vi "test cli options.vi"() -> ()   [LabVIEW 2024]
uses:
  <vilib>/Wiresmith Technology/G CLI/Argument Parser/Option Set Class/Option Set.lvclass
panel:
  out "help message":string
  out "Trailling Arguments":string[](array[string])
  out "files-to-include":string
  out "help set":bool
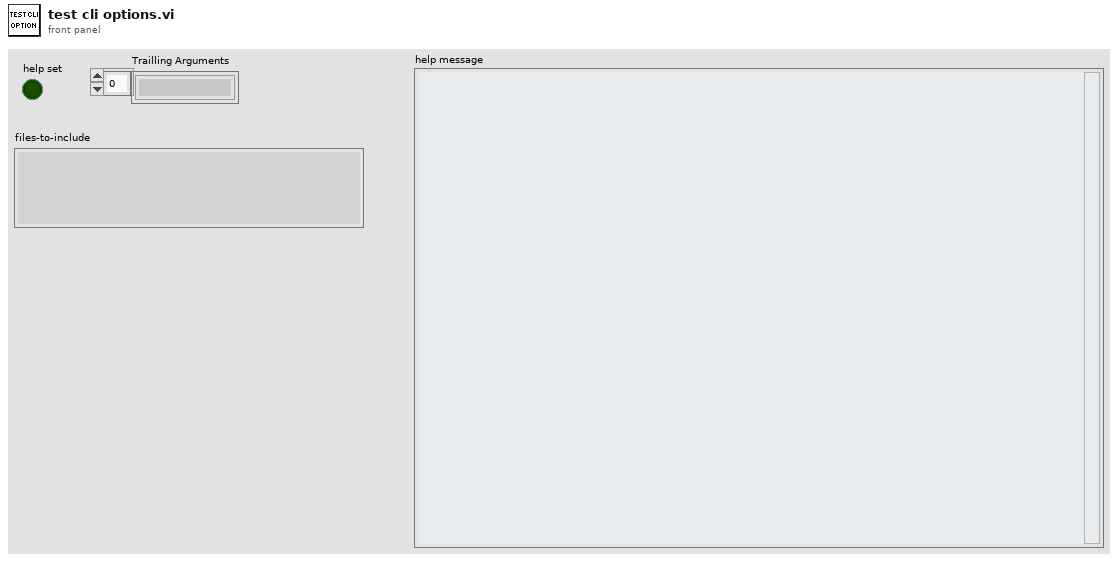
[diagram p1: front panel]
types:
  T1 = typedef "Option Parser.lvlib/Option.lvclass/Option Configuration.ctl" = cluster{"Option Type":T2, "Option Labels":string[], "Key":string, "Description":string, "Required":bool, "Default Value":string}
  T2 = typedef "Option Parser.lvlib/Option.lvclass/Argument Type.ctl" = enum16{"flag", "value"}
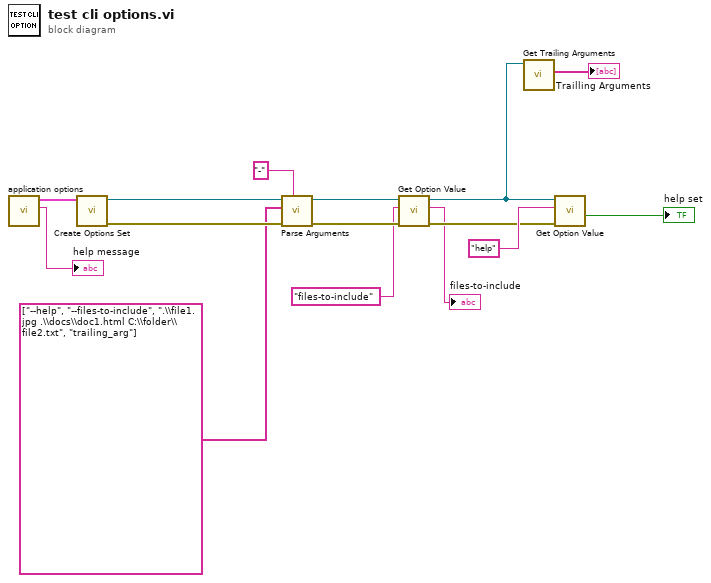
[diagram p0: block diagram]
diagram:
  n1 = call "application options.vi"() -> ("help message"=→"help message":string, "Options"=w9:T1[])  [unwired: 10 in]
  n2 = call <vilib>:"Create Options Set.vi"("Options"=w9) -> ("error out"=w14:errorcluster, "Option Set out"=w15:refnum<class "Option Set.lvclass">)  [unwired: 9 in]
  n3 = call <vilib>:"Parse Arguments.vi"("Label Marker (-)"="-", "error in (no error)"=w14, "Arguments"=string[] ["--help", "--files-to-include", ".\\file1.jpg .\\docs\\doc1.html C:\\folder\\file2.txt", "trailing_arg"], "Option Set in"=w15) -> ("error out"=w8:errorcluster, "Option Set out"=w6:refnum<class "Option Set.lvclass">)  [unwired: 4 in, 2 out]
  n4 = call <vilib>:"Get Option Value.vi"("error in (no error)"=w8, "Option Key"="files-to-include", "Option Set in"=w6) -> ("error out"=w7:errorcluster, "Value"=→"files-to-include":string, "Option Set out"=w3:refnum<class "Option Set.lvclass">)  [unwired: 5 in, 1 out]
  n5 = call <vilib>:"Get Trailing Arguments.vi"("Option Set in"=w3) -> ("Arguments"=→"Trailling Arguments":string[])  [unwired: 8 in, 2 out]
  n6 = call <vilib>:"Get Option Value.vi"("error in (no error)"=w7, "Option Key"="help", "Option Set in"=w3) -> ("Set"=→"help set":bool)  [unwired: 5 in, 3 out]
